vi "worksheet set h pagebreaks.vi"(8 "error in (no error)":errorcluster, 10 "breaks":u32, 11 "worksheet":u32) -> (0 "error out":errorcluster)   [LabVIEW 2015, in "xlsxwriter.lvlib"]
doc: "void worksheet_set_h_pagebreaks(lxw_worksheet worksheet, unsigned long breaks);"
uses:
  xlsxwriter.lvlib
  xlsxwriter.dll
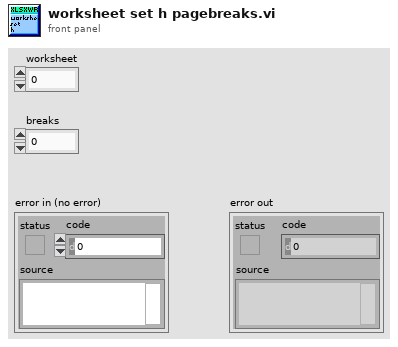
[diagram p1: front panel]
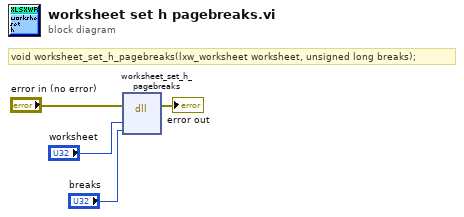
[diagram p0: block diagram]
diagram:
  # "void worksheet_set_h_pagebreaks(lxw_worksheet worksheet, unsigned long breaks);"
  n1 = dll-call lib="C:/Users/WDAGUtilityAccount/Desktop/lv_vis_added_cell/xlsxwriter.*" fn="worksheet_set_h_pagebreaks"(error in="error in (no error)", "worksheet"="worksheet", "breaks"="breaks") -> (error out=→"error out":errorcluster)  [unwired: 5 in, 1 out]
